vi "Acquire Temperature Data Value (Simulated).vi"() -> (0 "Thermometer":dbl(slide) scale=0.0..100.0)   [LabVIEW 2011]
doc: "This VI simulates acquiring temperature data one value at a time from a plug-in data acquisition board. The temperature is displayed in degrees Fahrenheit."
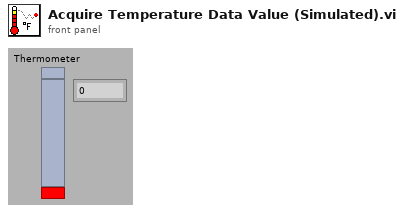
[diagram p1: front panel]
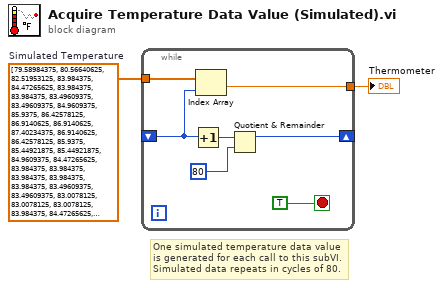
[diagram p0: block diagram]
diagram:
  w2 = dbl[] [79.58984375, 80.56640625, 82.51953125, 83.984375, 84.47265625, 83.984375, 83.984375, 83.49609375, 83.49609375, 84.9609375, 85.9375, 86.42578125, 86.9140625, 86.9140625, 87.40234375, 86.9140625, 86.42578125, 85.9375, 85.44921875, 85.44921875, 84.9609375, 84.47265625, 83.984375, 83.984375, 83.984375, 83.984375, 83.984375, 83.49609375, 83.49609375, 83.0078125, 83.0078125, 83.0078125, 83.984375, 84.47265625, 84.9609375, 85.44921875, 86.42578125, 86.9140625, 86.9140625, 86.9140625, 86.42578125, 85.9375, 85.44921875, 85.9375, 86.9140625, 87.40234375, 87.890625, 87.40234375, 86.9140625, 86.9140625, 85.9375, 85.9375, 85.9375, 84.9609375, 84.9609375, 84.9609375, 84.47265625, 84.47265625, 85.44921875, 85.9375, 86.9140625, 86.9140625, 86.42578125, 85.9375, 85.44921875, 85.44921875, 84.9609375, 84.9609375, 84.47265625, 84.47265625, 83.984375, 83.984375, 83.49609375, 83.49609375, 83.0078125, 83.0078125, 83.0078125, 83.0078125, 83.0078125, 83.0078125, 83.0078125, 82.51953125, 81.0546875, 81.54296875, 82.51953125, 83.0078125, 82.51953125, 82.03125, 82.03125, 82.03125, 82.03125, 81.54296875, 81.54296875, 81.54296875, 81.54296875]  # Simulated Temperature
  # "One simulated temperature data value \nis generated for each call to this subVI.  \nSimulated data repeats in cycles of 80."
  n1 = while {
    tunnel: w2 -> [w4]
    tunnel: [w5] -> w1
    shift-left: _ -> [w9]
    shift-right: [w6] -> _
    stop <- TRUE stop-if-true
    n2 = Increment(x=w9) -> (x+1=w8:i32)
    n3 = Index Array(array=w4, index=w9) -> (element=w5:dbl)
    n4 = Quotient & Remainder(x=w8, y=80) -> (x-y*floor(x/y)=w6:i32)  [unwired: 1 out]
  }
  "Thermometer" <- w1
